vi "Aircraft TX main.vi"(11 "Instance Details":T1) -> ()   [LabVIEW 2014]
uses:
  Ground Station to Aircraft Coms/SubVI/Aircraft Data Router/Controls/Known Aircraft.ctl
  Ground Station to Aircraft Coms/SubVI/Hardware Driver/Controls/Coms Driver Interface.ctl
  Telemetry/Controls/Telemetry Connection Type.ctl
  <vilib>/httpClient/ClientHandle.ctl
  Web Services/DronePi Global Variables.vi
  <vilib>/httpClient/LabVIEWHTTPClient.lvlib
panel:
  out "IP":string
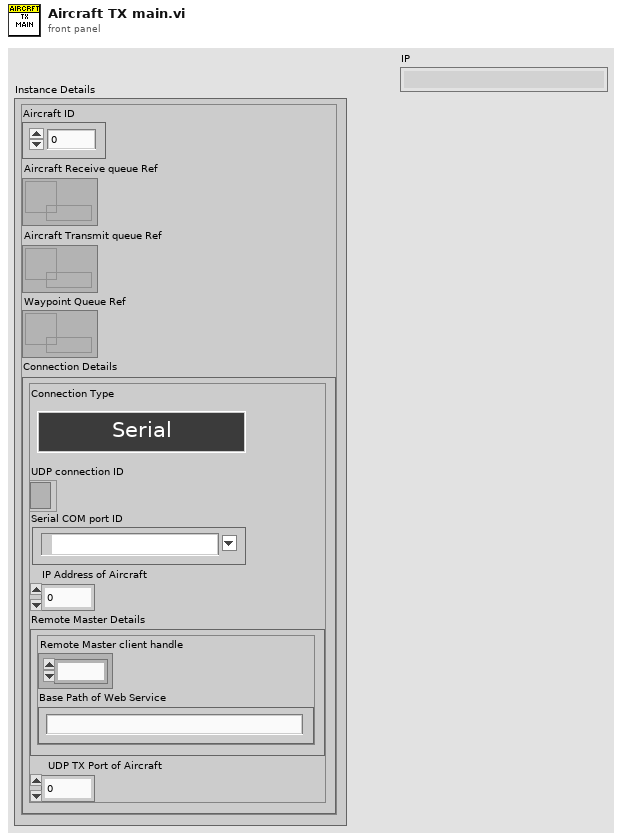
[diagram p1: front panel]
types:
  T1 = typedef "Known Aircraft.ctl" = cluster{"Aircraft ID":u8, "Aircraft Receive queue Ref":refnum<queue>, "Aircraft Transmit queue Ref":refnum<queue>, "Waypoint Queue Ref":refnum<queue>, "Connection Details":T2}
  T2 = typedef "Coms Driver Interface.ctl" = cluster{"Connection Type":T3, "UDP connection ID":refnum<k16>, "Serial COM port ID":refnum<visa-resource-name>, "IP Address of Aircraft":u32, "Remote Master Details":cluster{"Remote Master client handle":T4, "Base Path of Web Service":string}, "UDP TX Port of Aircraft":u16}
  T3 = typedef "Telemetry Connection Type.ctl" = enum16{"Serial", "UDP", "Remote Master"}
  T4 = typedef "LabVIEWHTTPClient.lvlib/ClientHandle.ctl" = refnum<k1>
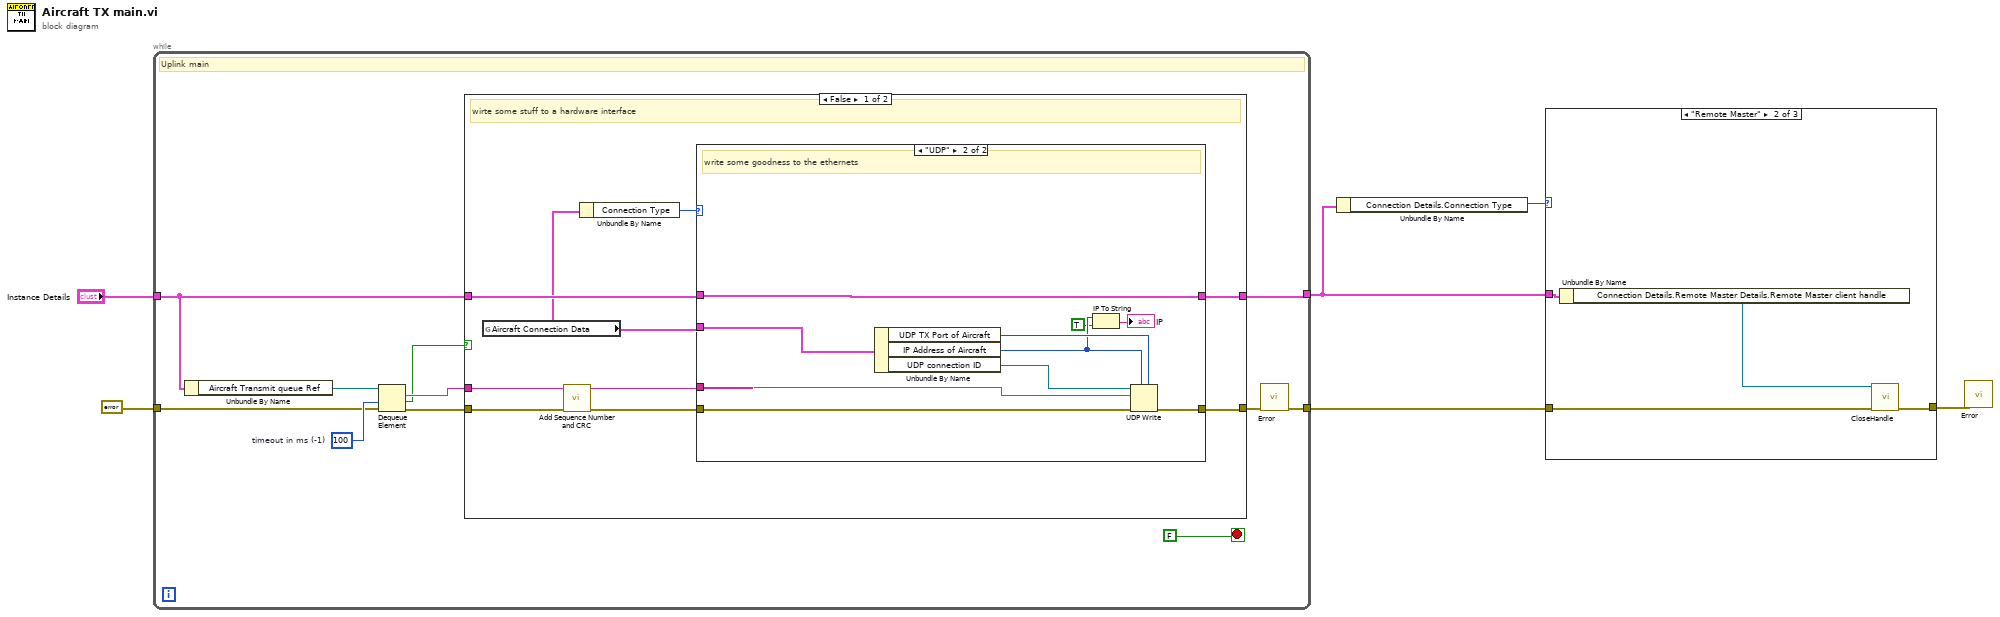
[diagram p0: block diagram]
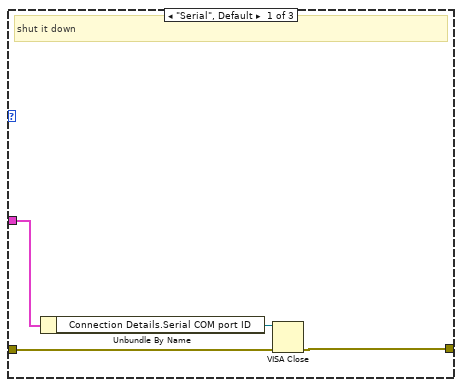
[diagram p2: hidden frame]
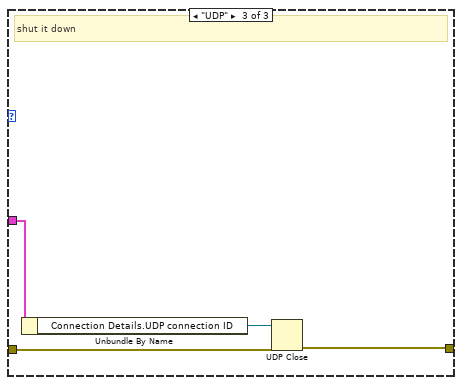
[diagram p3: hidden frame]
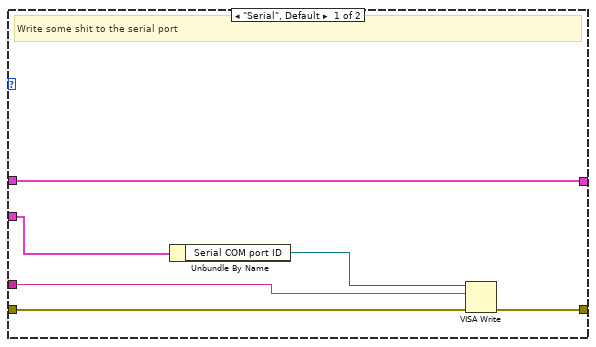
[diagram p4: hidden frame]
diagram:
  n1 = while {
    tunnel: errorcluster {"status"=FALSE, "code"=0, "source"=""} ("Error In") -> [w12]
    tunnel: [w8] -> w4
    tunnel: [w13] -> w5
    tunnel: "Instance Details" -> [w10]
    stop <- FALSE stop-if-true
    w15 = 100  # timeout in ms (-1)
    # "Uplink main"
    n2 = Unbundle By Name(w10) -> ("Aircraft Transmit queue Ref"=w11:refnum<queue>)
    n3 = Dequeue Element(queue=w11, timeout in ms (-1)=w15, error in (no error)=w12) -> (element=w17:string, timed out?=w14:bool, error out=w16:errorcluster)  [unwired: 1 out]
    n4 = case shown="False" w14 {
      tunnel: w17 -> [w25 _]
      tunnel: w16 -> [w24 w44]
      tunnel: [w26 w44] -> w9
      tunnel: w10 -> [w20 w43]
      tunnel: [w21 w43] -> w13
      frame False {
        # "wirte some stuff to a hardware interface"
        n5 = global read "DronePi Global Variables.vi" "Aircraft Connection Data"() -> (w18:T2)
        n6 = call "Add Sequence Number and CRC.vi"("Error In"=w24, "Message In"=w25) -> ("Error Out"=w22:errorcluster, "MAVLink Message Out"=w23:string)  [unwired: 8 in]
        n7 = Unbundle By Name(w18) -> ("Connection Type"=w19:T3)
        n8 = case shown="\"UDP\"" w19 {
          tunnel: w23 -> [w29 w40]
          tunnel: [w32 w39] -> w26
          tunnel: w22 -> [w31 w42]
          tunnel: w20 -> [w28 w34]
          tunnel: [w28 w34] -> w21
          tunnel: w18 -> [w27 w33]
          frame "Serial", Default {
            # "Write some shit to the serial port"
            n9 = Unbundle By Name(w27) -> ("Serial COM port ID"=w30:refnum<visa-resource-name>)
            n10 = VISA Write(VISA resource name=w30, write buffer=w29, error in (no error)=w31) -> (error out=w32:errorcluster)  [unwired: 2 out]
          }
          frame "UDP" {
            # "write some goodness to the ethernets"
            n11 = Unbundle By Name(w33) -> ("UDP TX Port of Aircraft"=w38:u16, "IP Address of Aircraft"=w37:u32, "UDP connection ID"=w41:refnum<k16>)
            n12 = IP To String(1:TRUE ("dot notation? (F)"), 2:w37) -> (0:→"IP":string)
            n13 = UDP Write(address=w37, port or service name=w38, connection ID=w41, data in=w40, 8:w42) -> (error out=w39:errorcluster)  [unwired: 1 in, 1 out]
          }
        }
      }
      frame True {
        # "Timed out. do nothing"
      }
    }
    n14 = call "Error.vi"("Error In"=w9) -> ("Error Out"=w8:errorcluster)  [unwired: 10 in]
  }
  n15 = Unbundle By Name(w5) -> ("Connection Details.Connection Type"=w6:T3)
  n16 = case shown="\"Remote Master\"" w6 {
    tunnel: [w48 w50 w55] -> w3
    tunnel: w4 -> [w47 w51 w53]
    tunnel: w5 -> [w46 w52 w56]
    frame "Serial", Default {
      # "shut it down"
      n17 = Unbundle By Name(w46) -> ("Connection Details.Serial COM port ID"=w45:refnum<visa-resource-name>)
      n18 = VISA Close(VISA resource name=w45, error in (no error)=w47) -> (error out=w48:errorcluster)
    }
    frame "Remote Master" {
      n19 = Unbundle By Name(w52) -> ("Connection Details.Remote Master Details.Remote Master client handle"=w49:T4)
      n20 = call <vilib>:"CloseHandle.vi"("client handle"=w49, "error in (no error)"=w51) -> ("error out"=w50:errorcluster)  [unwired: 13 in]
    }
    frame "UDP" {
      # "shut it down"
      n21 = Unbundle By Name(w56) -> ("Connection Details.UDP connection ID"=w54:refnum<k16>)
      n22 = UDP Close(connection ID=w54, 8:w53) -> (error out=w55:errorcluster)  [unwired: 1 out]
    }
  }
  n23 = call "Error.vi"("Error In"=w3) -> ()  [unwired: 10 in, 1 out]
